vi "_DelEmptRow (SubVI).vi"(11 "all rows in":string[][](array[string])) -> (3 "all rows out":string[][](array[string]))   [LabVIEW 2017]
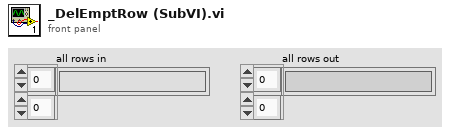
[diagram p1: front panel]
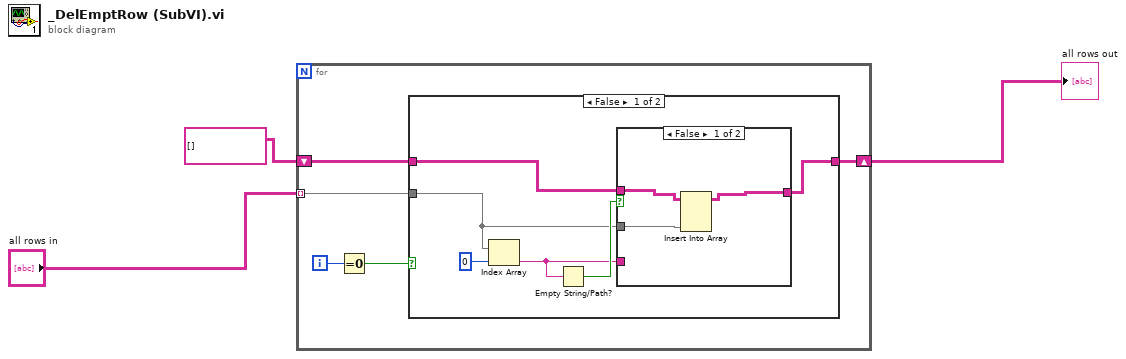
[diagram p0: block diagram]
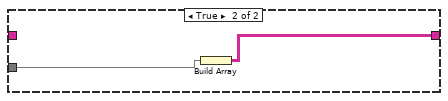
[diagram p3: hidden frame]
diagram:
  n1 = for {
    tunnel: "all rows in" -> [w7] mode=indexing
    shift-right: [w6] -> w3
    shift-left: string[][] [] ("all rows") -> [w8]
    i -> [w5]
    n2 = Equal To 0?(x=w5) -> (x = 0?=w4:bool)
    n3 = case shown="False" w4 {
      tunnel: w8 -> [w14 _]
      tunnel: w7 -> [w9 w20]
      tunnel: [w11 w19] -> w6
      frame False {
        n4 = Index Array(array=w9, index=0) -> (element=w10:string)
        n5 = Empty String/Path?(string/path=w10) -> (empty?=w12:bool)
        n6 = case shown="False" w12 {
          tunnel: w14 -> [w17 w18]
          tunnel: [w16 w18] -> w11
          tunnel: w10 -> [_ _]
          tunnel: w9 -> [w15 _]
          frame False {
            n7 = Insert Into Array(array=w17, new element=w15) -> (w16:string[][])  [unwired: 2 in]
          }
          frame True {
          }
        }
      }
      frame True {
        n8 = Build Array(w20) -> (w19:string[][])
      }
    }
  }
  "all rows out" <- w3
